vi "xijk_select_best_filter_sort.vi"(5 "Column Sort Order":i32[](array[numeric]), 6 "Preview Sorted Data? (F)":bool, 7 "Output Columns in Sort Order? (F)":bool, 8 "Calling VI Name":string, 9 "Sort Ascending? (T)":T1, 10 "Input Array Contains Header Row? (T)":T2, 11 "Input Array":string[][](array[string])) -> (3 "Output Array":string[][](array[string]))   [LabVIEW 2009, in "xijk_select_best_filter.lvlib"]
uses:
  xijk_select_best_filter.lvlib
  Sorting/_TypeDefs/TYPE - Input Array Contains Header Row.ctl
  Sorting/_TypeDefs/TYPE - Sort Ascending.ctl
panel:
  out "Sorted Array":string[][](table)
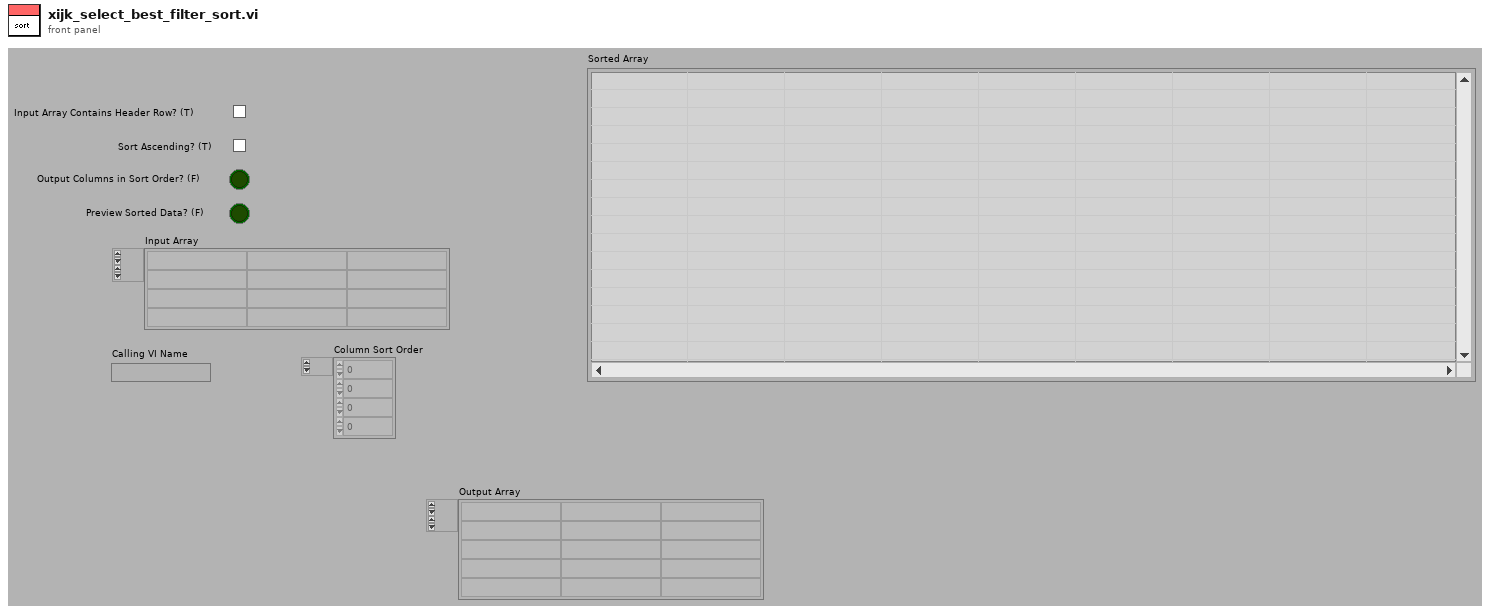
[diagram p1: front panel]
types:
  T1 = typedef "xijk_select_best_filter.lvlib/TYPE - Sort Ascending.ctl" = bool
  T2 = typedef "xijk_select_best_filter.lvlib/TYPE - Input Array Contains Header Row.ctl" = bool
  T3 = typedef "xijk_select_best_filter.lvlib/TYPE - Sorted Array (Cols in Original Order. Header row removed).ctl" = string[][]
  T4 = typedef "xijk_select_best_filter.lvlib/TYPE - Sorted Array (Cols in Sort Order. Header row removed).ctl" = string[][]
  T5 = typedef "xijk_select_best_filter.lvlib/TYPE - Sorted Array (Cols in Sort Order. Headers as last row).ctl" = string[][]
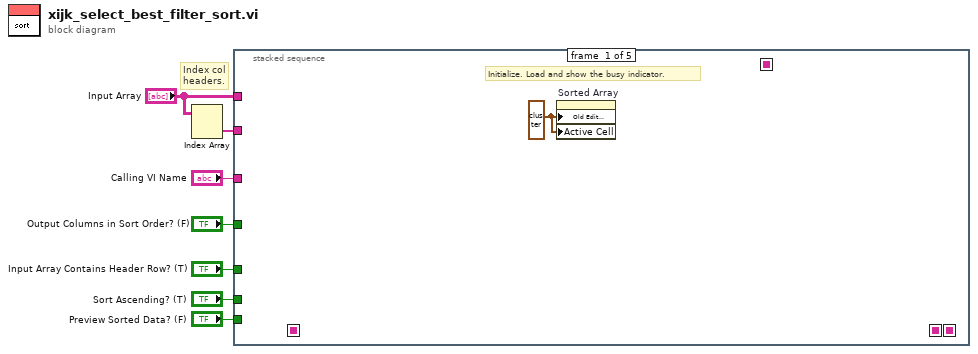
[diagram p0: block diagram]
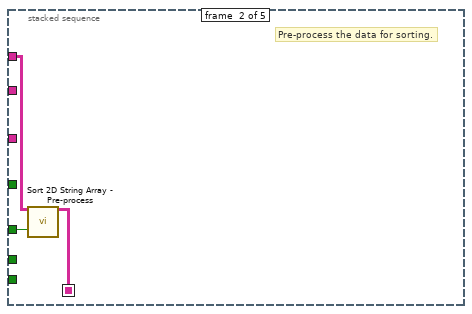
[diagram p2: hidden frame]
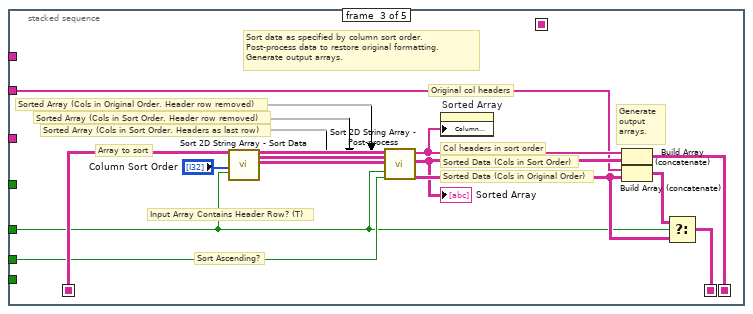
[diagram p3: hidden frame]
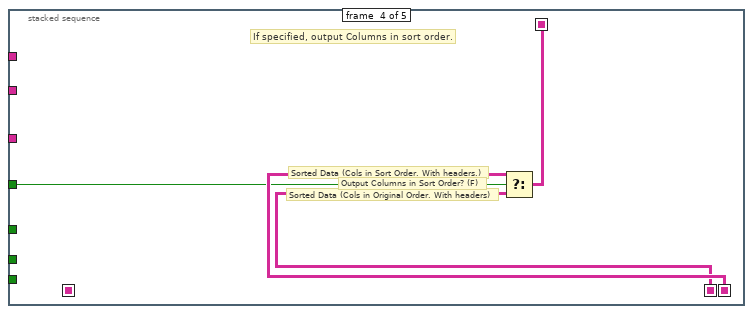
[diagram p4: hidden frame]
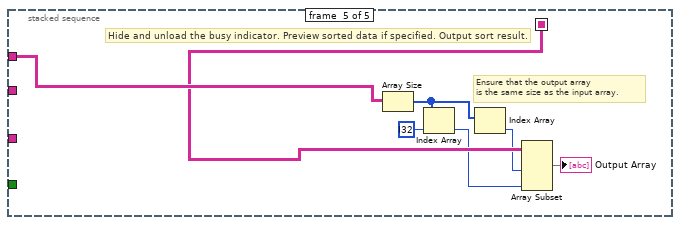
[diagram p5: hidden frame]
diagram:
  # "Index col\nheaders."
  n1 = Index Array(array="Input Array") -> (element=w3:string[])  [unwired: 2 in]
  n2 = stacked-sequence {
    seq-local: [_ w9 _ _ _] -> [_ _ w21 _ _]
    seq-local: [_ _ w15 _ _] -> [_ _ _ w28 _]
    seq-local: [_ _ w20 _ _] -> [_ _ _ w29 _]
    seq-local: [_ _ _ w26 _] -> [_ _ _ _ w35]
    tunnel: "Input Array" -> [_ w11 _ _ w36]
    tunnel: "Input Array Contains Header Row? (T)" -> [_ w10 w12 _ _]
    tunnel: w3 -> [_ _ w13 _ _]
    tunnel: "Sort Ascending? (T)" -> [_ _ w19 _ _]
    tunnel: "Output Columns in Sort Order? (F)" -> [_ _ _ w27 _]
    tunnel: "Preview Sorted Data? (F)" -> [_ _ _ _ _]
    tunnel: "Calling VI Name" -> [_ _ _ _ _]
    frame #0 {
      w8 = cluster{i32, i32} ? ("Write Attribute")
      # "Initialize. Load and show the busy indicator."
      n3 = property on="Sorted Array" class="Tbl (strict)"("Old Edit Position"=w8, "Active Cell"=w8) -> ()  [unwired: 2 in, 2 out]
    }
    frame #1 {
      # "Pre-process the data for sorting."
      n4 = call "Sort 2D String Array - Pre-process.vi"("Array to Sort In"=w11, "Input Array Contains Header Row? (T)"=w10) -> ("Array to Sort Out"=w9:string[][])  [unwired: 1 in, 16 out]
    }
    frame #2 {
      # "Sort Ascending?"
      # "Generate\noutput\narrays."
      # "Sort data as specified by column sort order.\nPost-process data to restore original formatting.\nGenerate output arrays."
      # "Original col headers"
      # "Input Array Contains Header Row? (T)"
      # "Sorted Array (Cols in Original Order. Header row removed)"
      # "Sorted Array (Cols in Sort Order. Header row removed)"
      # "Sorted Array (Cols in Sort Order. Headers as last row)"
      # "Sorted Data (Cols in Original Order)"
      # "Sorted Data (Cols in Sort Order)"
      # "Col headers in sort order"
      # "Array to sort"
      n5 = call "Sort 2D String Array - Sort Data.vi"("Array to sort in"=w21, "Column Sort Order"="Column Sort Order", "Input Array Contains Header Row? (T)"=w12) -> ("Sorted Array (Cols in Original Order. Header row removed)"=w22:T3, "Sorted Array (Cols in Sort Order. Header row removed)"=w25:T4, "Sorted Array (Cols in Sort Order. Headers as last row)"=w24:T5)  [unwired: 6 in, 8 out]
      n6 = call "Sort 2D String Array - Post-process.vi"("Sorted Array (Cols in Original Order. Header row removed)"=w22, "Sorted Array (Cols in Sort Order. Header row removed)"=w25, "Sorted Array (Cols in Sort Order. Headers as last row)"=w24, "Input Array Contains Header Row? (T)"=w12, "Sort Ascending? (T)"=w19) -> ("Column Headers (In Sort Order)"=w18:string[], "Sorted Data (Columns in Sort Order)"=w14:string[][], "Sorted Data (Columns in Original Order)"=w17:string[][])  [unwired: 5 in, 7 out]
      "Sorted Array" <- w14
      n7 = property on="Sorted Array" class="Tbl (strict)"("Column Headers[]"=w18) -> ()  [unwired: 2 in, 2 out]
      n8 = Build Array (concatenate)(w18, w14) -> (w20:string[][])
      n9 = Build Array (concatenate)(w13, w17) -> (w16:string[][])
      n10 = Select(t=w16, s=w12, f=w17) -> (s? t:f=w15:string[][])
    }
    frame #3 {
      # "If specified, output Columns in sort order."
      # "Sorted Data (Cols in Original Order. With headers)"
      # "Sorted Data (Cols in Sort Order. With headers.)"
      # "Output Columns in Sort Order? (F)"
      n11 = Select(t=w29, s=w27, f=w28) -> (s? t:f=w26:string[][])
    }
    frame #4 {
      # "Ensure that the output array\nis the same size as the input array."
      # "Hide and unload the busy indicator. Preview sorted data if specified. Output sort result."
      n12 = Array Size(array=w36) -> (size(s)=w33:i32[])
      n13 = Index Array(array=w33, index=i32 ?) -> (element=w30:i32)
      n14 = Index Array(array=w33) -> (element=w31:i32)  [unwired: 1 in]
      n15 = Array Subset(array=w35, length (row)=w31, length (col)=w30) -> (→"Output Array":string[][])  [unwired: 2 in]
    }
  }
